vi "Write configuration.vi"(8 "error in (no error)":errorcluster, 11 "Cascade512II in":refnum<class "DAQCascade512II.lvclass">) -> (0 "error out":errorcluster, 3 "Cascade512II out":refnum<class "DAQCascade512II.lvclass">)   [LabVIEW 2012, in "DAQCascade512II.lvclass"]
doc: "Writes the configuration cluster into the configuration file. Configuration file is XML-based. It's name is <component ID>.xml"
uses:
  DAQCascade512II.lvclass
  <vilib>/Distrio/Murmex/Murmex/Murmex.lvclass
  DAQCascade512II.lvclass/DAQCascade512II.ctl
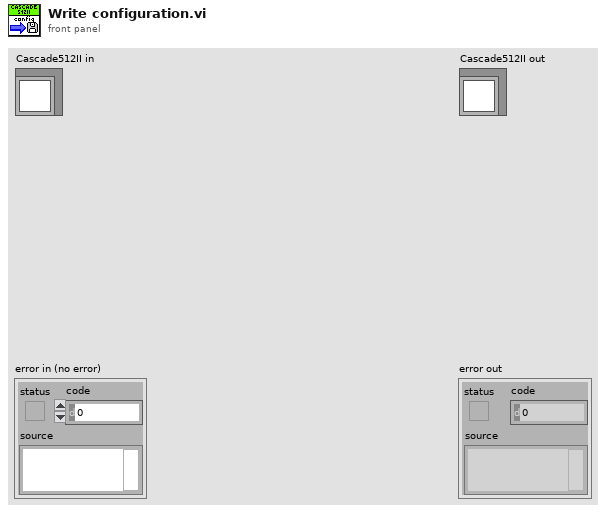
[diagram p1: front panel]
types:
  T1 = typedef "DAQCascade512II.lvclass/configuration cluster.ctl" = cluster{"Temperature":dbl, "Acquire / Focus Flag  of trigger":u32, "Number of Images fo Initializer":u32, "Data Type":u32, "Timing Mode of trigger ":u32, "Gain multiplication":dbl, "Fast ADC":bool}
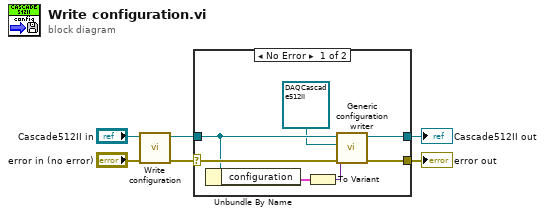
[diagram p0: block diagram]
diagram:
  n1 = call-parent "Write configuration.vi"("error in (no error)"="error in (no error)", "Murmex in"="Cascade512II in") -> ("error out"=w4:errorcluster, "Murmex out"=w2:refnum<class "DAQCascade512II.lvclass">)  [unwired: 8 in]
  n2 = case shown="No Error" w4 {
    selector: w4 -> [w13 w14]
    tunnel: [w12 w14] -> w3
    tunnel: w2 -> [w10 w15]
    tunnel: [w11 w15] -> w1
    frame No Error {
      n3 = Unbundle By Name(w10) -> ("configuration"=w9:T1)
      n4 = To Variant(anything=w9) -> (Variant=w8:variant)
      n5 = call <vilib>:"Generic configuration writer.vi"("error in (no error)"=w13, "configuration"=w8, "inheritance level"=refnum<class "DAQCascade512II.lvclass"> refnum ("DAQCascade512II"), "MurmexBase in"=w10) -> ("error out"=w12:errorcluster, "MurmexBase out"=w11:refnum<class "DAQCascade512II.lvclass">)  [unwired: 6 in]
    }
    frame Error {
    }
  }
  "error out" <- w3
  "Cascade512II out" <- w1
